vi "REWORK_display_messages_history.vi"(8 "error_in":errorcluster) -> (0 "error_out":errorcluster)   [LabVIEW 2019]
uses:
  FGV_REWORK_DIAGNOSTICS_message_history_display.ctl
  FGV/DIAGNOSTICS_message_history_buffer/FGV_REWORK_DIAGNOSTICS_message_history_buffer.ctl
  _misc/AULocalize/SubVIs/RegisterVI.vi
panel:
  out "Message History":string caption="(ий)Message History"
  in  "clear_messages":bool
  in  "STOP":bool
  in  "refresh_messages":bool
  in  "messages_history_lbx":i32(listbox)
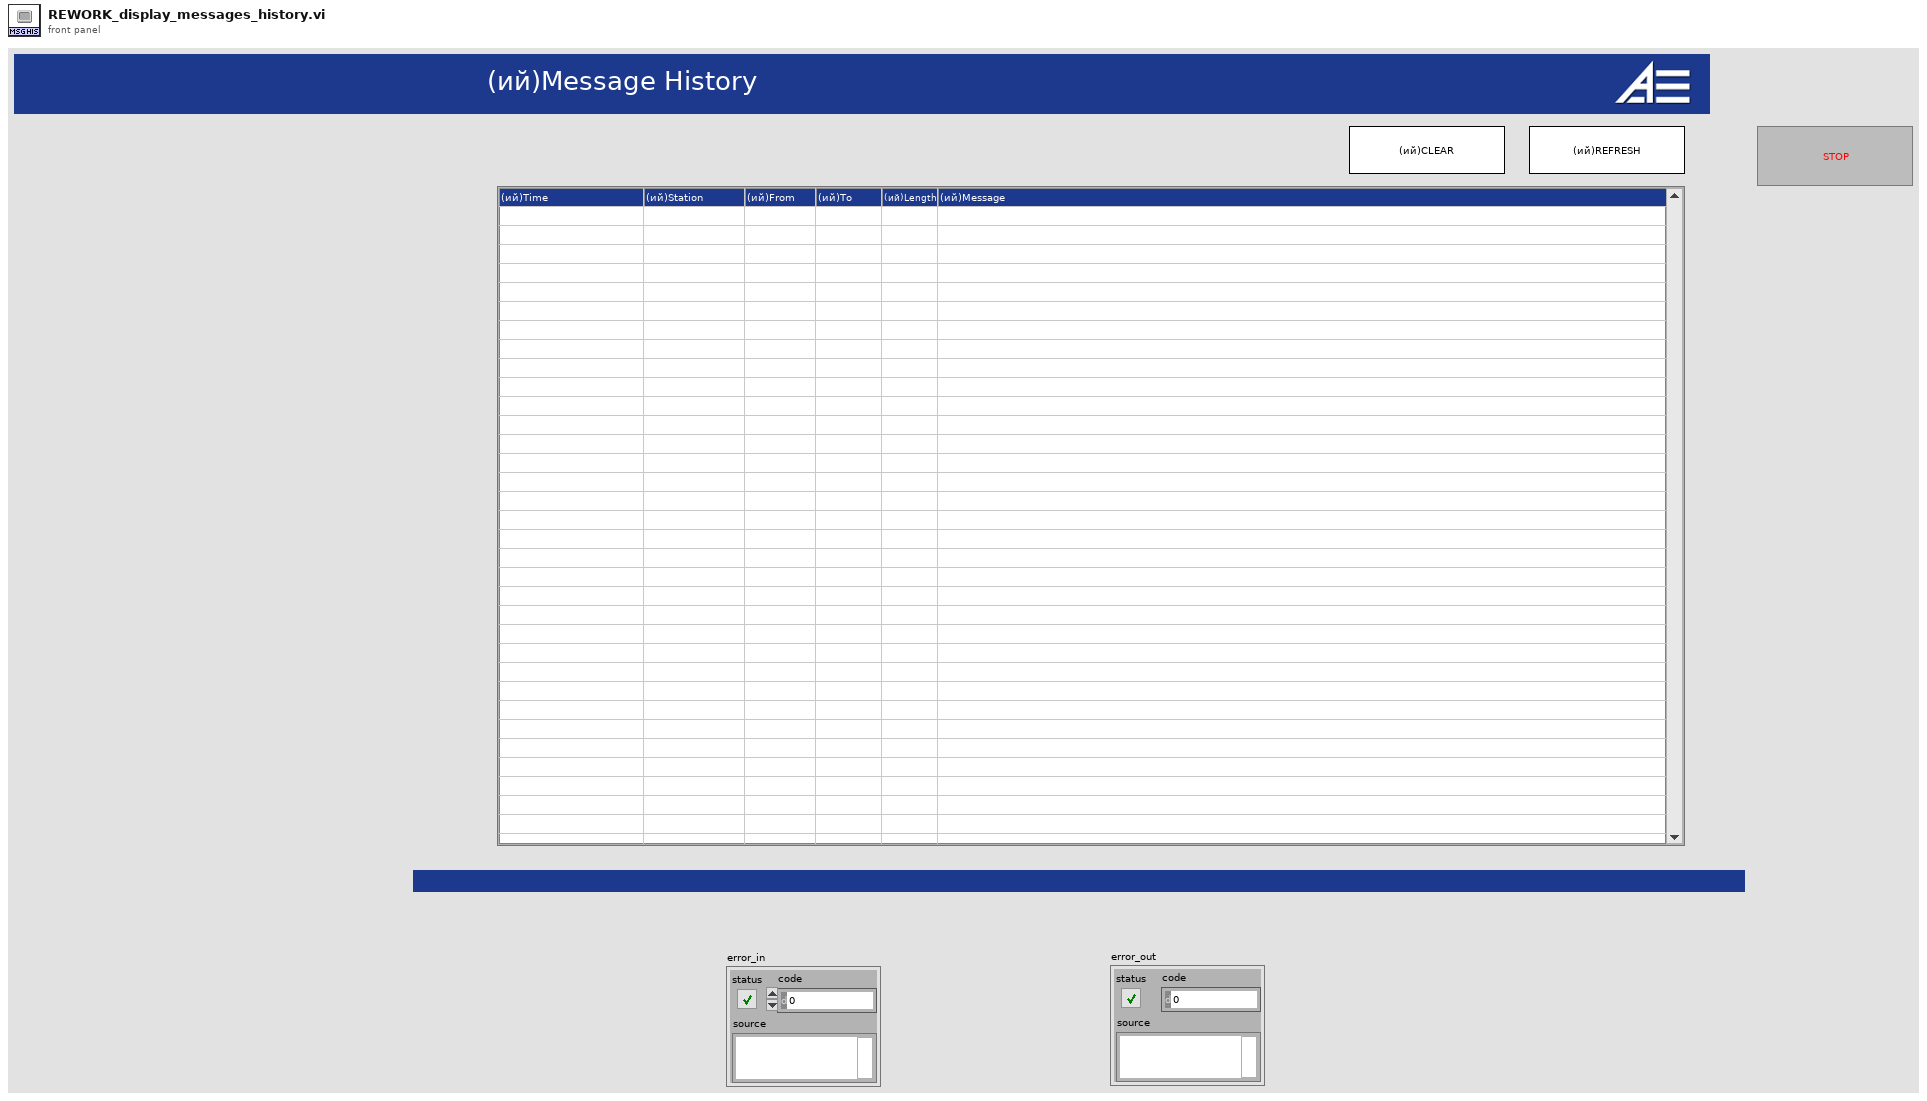
[diagram p1: front panel]
types:
  T1 = typedef "FGV_REWORK_DIAGNOSTICS_message_history_buffer.ctl" = enum16{"initialize", "add_TCP_PLC_to_PC", "add_TCP_PC_to_PLC", "add_SQL_PC_to_DB", "add_SQL_transaction", "add_SQL_DB_to_PC", "get_all", "clear_all", "save_log"}
  T2 = typedef "FGV_REWORK_DIAGNOSTICS_message_history_display.ctl" = enum16{"initialize", "display_messages"}
  T3 = typedef "REWORK_DIAGNOSTICS_message_history_buffer_all_info.ctl" = cluster{"timestamp":timestamp, "message_type":T4, "message":string, "record":string[]}
  T4 = typedef "DIAGNOSTICS_message_type.ctl" = enum16{"TCP", "SQL"}
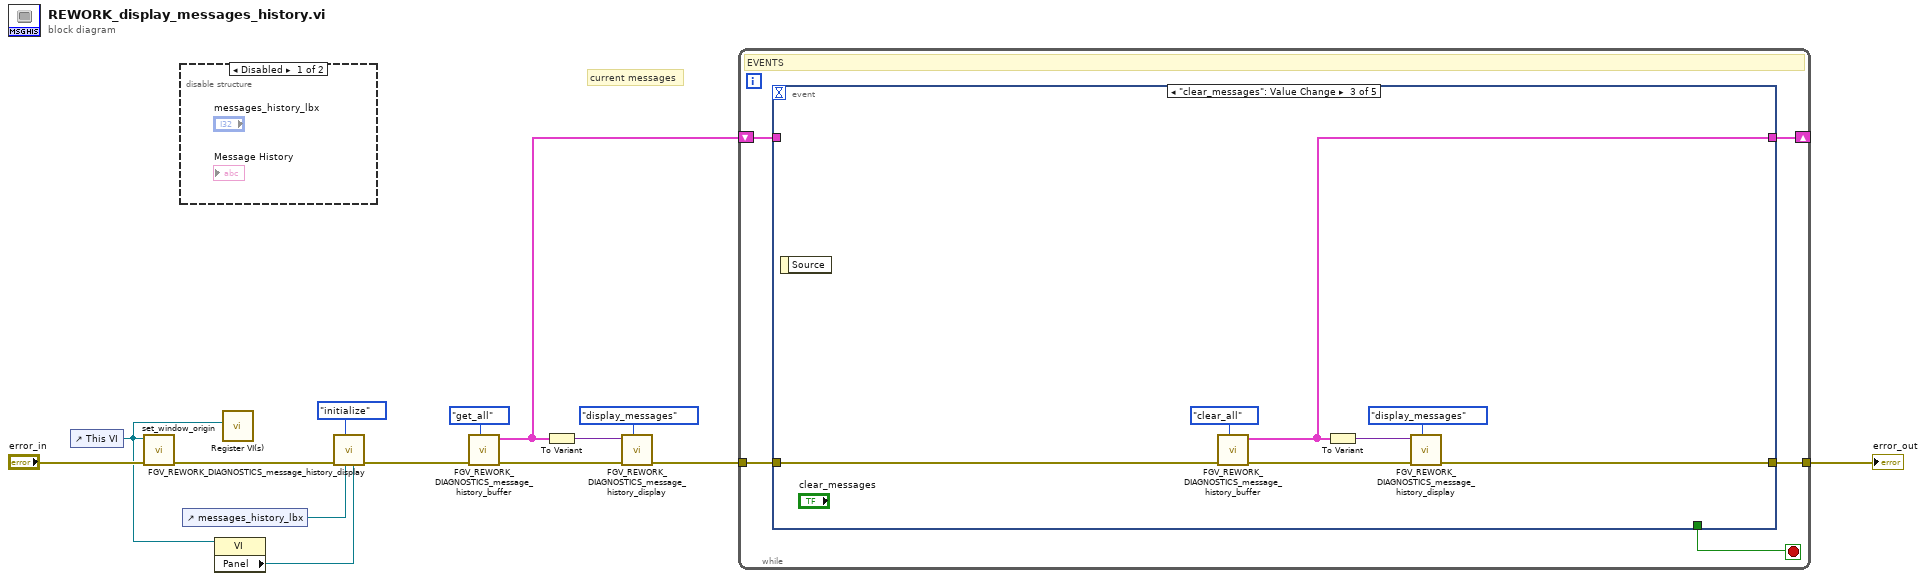
[diagram p0: block diagram]
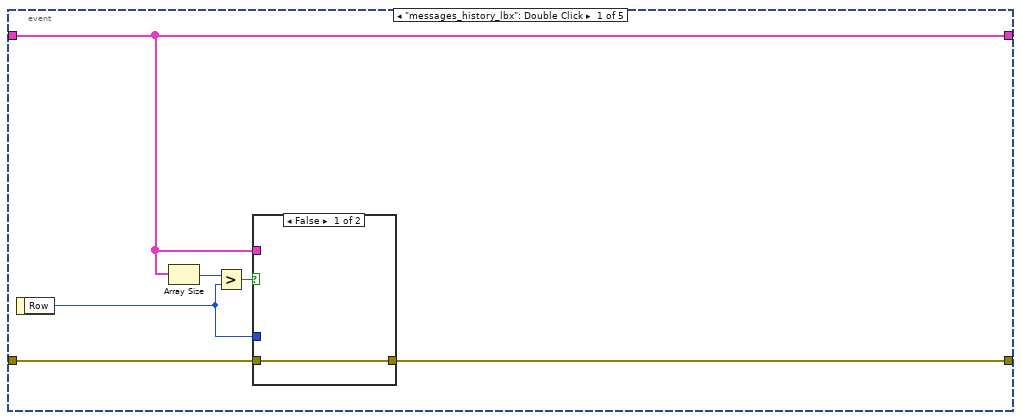
[diagram p3: hidden frame]
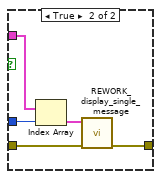
[diagram p4: hidden frame]
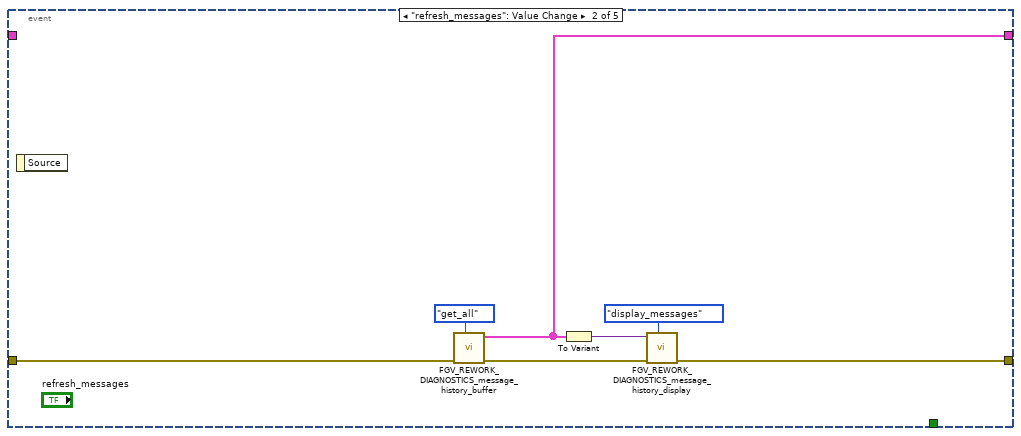
[diagram p5: hidden frame]
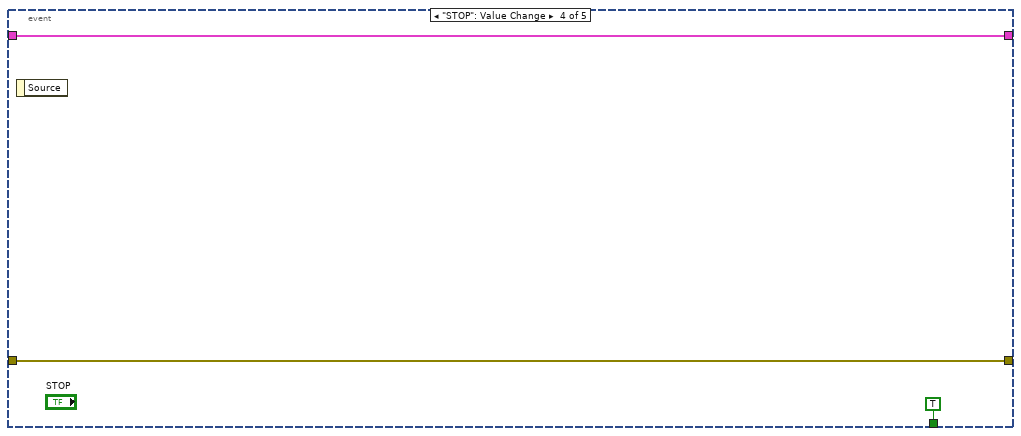
[diagram p6: hidden frame]
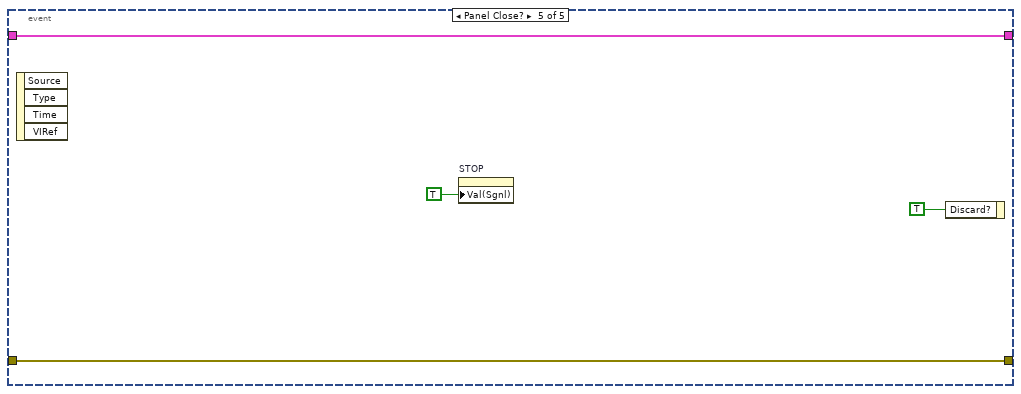
[diagram p7: hidden frame]
diagram:
  # "current messages"
  n1 = control-ref of="This VI"() -> (w1:refnum<vi>)
  n2 = call "set_window_origin.vi"("error_in"="error_in", "this_vi_reference"=w1) -> ("error_out"=w14:errorcluster)  [unwired: 9 in]
  n3 = disable-structure shown="Disabled" {
    frame Disabled {
    }
    frame Enabled {
    }
  }
  n4 = control-ref of="messages_history_lbx"() -> (w12:refnum<vi>)
  n5 = property class="VI"(reference=w1) -> ("Panel"=w13:refnum<vi>)  [unwired: 1 in, 2 out]
  n6 = call-poly "Register VI(s).vi"("VI Ref"=w1) -> ()  [unwired: 9 in, 2 out]
  n7 = call "FGV_REWORK_DIAGNOSTICS_message_history_display.vi"("front_panel_reference"=w13, "SQL_listbox_reference"=w12, "options"=FGV_REWORK_DIAGNOSTICS_message_history_display."initialize", "error_in"=w14) -> ("error_out"=w4:errorcluster)  [unwired: 7 in]
  n8 = call "FGV_REWORK_DIAGNOSTICS_message_history_buffer.vi"("options"=FGV_REWORK_DIAGNOSTICS_message_history_buffer."get_all", "error_in"=w4) -> ("error_out"=w3:errorcluster, "message_history"=w2:T3[])  [unwired: 8 in]
  n9 = To Variant(anything=w2) -> (Variant=w6:variant)
  n10 = call "FGV_REWORK_DIAGNOSTICS_message_history_display.vi"("options"=FGV_REWORK_DIAGNOSTICS_message_history_display."display_messages", "error_in"=w3, "input"=w6) -> ("error_out"=w5:errorcluster)  [unwired: 8 in]
  n11 = while {
    tunnel: [w19] -> w11
    tunnel: w5 -> [w17]
    shift-right: [w16] -> _
    shift-left: w2 -> [w15]
    stop <- w18 stop-if-true
    # "EVENTS"
    n12 = event shown="[2] \"clear_messages\": Value Change" {
      selector: _ -> [_ _ _ _ _]
      dyn-events: _ -> [_ _ _ _ _]
      timeout: _ -> [_ _ _ _ _]
      tunnel: [_ _ _ TRUE _] -> w18
      tunnel: w17 -> [w25 w38 w45 w48 w52]
      tunnel: [w24 w36 w43 w48 w52] -> w19
      tunnel: [w23 w33 w40 w46 w49] -> w16
      tunnel: w15 -> [w23 _ _ w46 w49]
      event "messages_history_lbx": Double Click {
        n13 = event-data() -> ("Row"=w21:i32)  [unwired: 1 in]
        n14 = Array Size(array=w23) -> (size(s)=w22:i32)
        n15 = Greater?(x=w22, y=w21) -> (0:w20:bool)
        n16 = case shown="False" w20 {
          tunnel: w25 -> [w26 w31]
          tunnel: [w26 w30] -> w24
          tunnel: w23 -> [_ w28]
          tunnel: w21 -> [_ w27]
          frame False {
          }
          frame True {
            n17 = Index Array(array=w28, index=w27) -> (element=w29:T3)
            n18 = call "REWORK_display_single_message.vi"("error_in"=w31, "message_history_buffer_element"=w29) -> ("error_out"=w30:errorcluster)  [unwired: 9 in]
          }
        }
      }
      event "refresh_messages": Value Change {
        n19 = event-data() -> ()  [unwired: 1 in, 1 out]
        n20 = call "FGV_REWORK_DIAGNOSTICS_message_history_buffer.vi"("options"=FGV_REWORK_DIAGNOSTICS_message_history_buffer."get_all", "error_in"=w38) -> ("error_out"=w37:errorcluster, "message_history"=w33:T3[])  [unwired: 8 in]
        n21 = To Variant(anything=w33) -> (Variant=w35:variant)
        n22 = call "FGV_REWORK_DIAGNOSTICS_message_history_display.vi"("options"=FGV_REWORK_DIAGNOSTICS_message_history_display."display_messages", "error_in"=w37, "input"=w35) -> ("error_out"=w36:errorcluster)  [unwired: 8 in]
      }
      event "clear_messages": Value Change {
        n23 = event-data() -> ()  [unwired: 1 in, 1 out]
        n24 = call "FGV_REWORK_DIAGNOSTICS_message_history_buffer.vi"("options"=FGV_REWORK_DIAGNOSTICS_message_history_buffer."clear_all", "error_in"=w45) -> ("error_out"=w44:errorcluster, "message_history"=w40:T3[])  [unwired: 8 in]
        n25 = To Variant(anything=w40) -> (Variant=w42:variant)
        n26 = call "FGV_REWORK_DIAGNOSTICS_message_history_display.vi"("options"=FGV_REWORK_DIAGNOSTICS_message_history_display."display_messages", "error_in"=w44, "input"=w42) -> ("error_out"=w43:errorcluster)  [unwired: 8 in]
      }
      event "STOP": Value Change {
        n27 = event-data() -> ()  [unwired: 1 in, 1 out]
      }
      event Panel Close? {
        n28 = event-data() -> ()  [unwired: 1 in, 4 out]
        n29 = property on="STOP" class="Bool (strict)"("Val(Sgnl)"=TRUE ("Value (Signaling)")) -> ()  [unwired: 2 in, 2 out]
        n30 = event-data("Discard?"=TRUE) -> ()  [unwired: 1 in, 1 out]
      }
    }
  }
  "error_out" <- w11
